vi "Autonomous Independent.vi"   [LabVIEW 2023]
doc: "This VI is called when autonomous begins, and will automatically be terminated when autonomous ends. You can carry out timed or sensor driven robot movement independently without needing to return to the caller."
uses:
  Auto states.ctl
  <vilib>/Rock Robotics/WPI/ThirdParty/REV Robotics/REVLib/Typedef/Spark MAX Idle Mode.ctl
  <vilib>/Rock Robotics/WPI/Utilities/WPI_GetSetVariantRefNum.vi
  <vilib>/Rock Robotics/Network Tables/NT Read String.vi
  <vilib>/Rock Robotics/Network Tables/NT Write Numeric Array.vi
  <vilib>/Rock Robotics/WPI/RobotDrive/WPI_RobotDriveArcadeDrive_Standard(NoSaturation).vi
panel:
  # "Be sure to right-click and choose Data Operations>>Make Current Value default if you want to save the array values with the VI"
types:
  T1 = typedef "WPI_JoystickDevRef.ctl" = cluster{"Device":T2}
  T2 = typedef "WPI_JoystickDeviceEnum.ctl" = enum16{"USB 0", "USB 1", "USB 2", "USB 3", "USB 4", "USB 5"}
  T3 = typedef "Auto states.ctl" = enum16{"Aim", "Fire", "Cross Line", "Pickup", "Reverse Intake", "Return", "Aim 2", "Fire 2", "End"}
  T4 = typedef "Spark MAX Idle Mode.ctl" = enum16{"Coast", "Brake"}
  T5 = typedef "WPI_MotorControlDeviceRef.ctl" = cluster{"DeviceStatus":errorcluster, "Type":T6, "PWM":cluster{"PWM Channel":T7, "DeadBand":T8}, "CAN":cluster{"Device Number":u8, "SetOutput VI Ref":variant, "GetOutput VI Ref":variant, "Enable VI Ref":variant, "Disable VI Ref":variant, "Data":variant}, "Invert":bool, "DIO PWM":cluster{"PWM \"Enable\" Channel":T7, "DIOChannel":T9, "PWM Rate":dbl}}
  T6 = typedef "WPI_MotorControlType.ctl" = enum16{"PWM", "CAN", "DIO PWM"}
  T7 = typedef "FPGA_DIOPWMChannel.ctl" = enum8{"PWM 0", "PWM 1", "PWM 2", "PWM 3", "PWM 4", "PWM 5", "PWM 6", "PWM 7", "PWM 8", "PWM 9", "PWM MXP 0", "PWM MXP 1", "PWM MXP 2", "PWM MXP 3", "PWM MXP 4", "PWM MXP 5", "PWM MXP 6", "PWM MXP 7", "PWM MXP 8", "PWM MXP 9", "Invalid"}
  T8 = typedef "WPI_PWMDeadband.ctl" = cluster{"Name":string, "maxPositivePwm":i32, "minPositivePwm":i32, "centerPwm":i32, "maxNegativePwm":i32, "minNegativePwm":i32, "angularRange":u16}
  T9 = typedef "FPGA_DIOChannel.ctl" = enum8{"DIO 0", "DIO 1", "DIO 2", "DIO 3", "DIO 4", "DIO 5", "DIO 6", "DIO 7", "DIO 8", "DIO 9", "DIO MXP 0", "DIO MXP 1", "DIO MXP 2", "DIO MXP 3", "DIO MXP 4", "DIO MXP 5", "DIO MXP 6", "DIO MXP 7", "DIO MXP 8", "DIO MXP 9", "DIO MXP 10", "DIO MXP 11", "DIO MXP 12", "DIO MXP 13", "DIO MXP 14", "DIO MXP 15", "SPI Port CS1", "SPI Port CS2", "SPI Port CS3", "SPI Port MISO", "SPI Port MOSI", "Invalid"}
  T10 = typedef "WPI_RobotDriveDevRef.ctl" = cluster{"DevStatus":errorcluster, "Motors[]":T5[], "Square Inputs":bool, "Max Output":dbl}
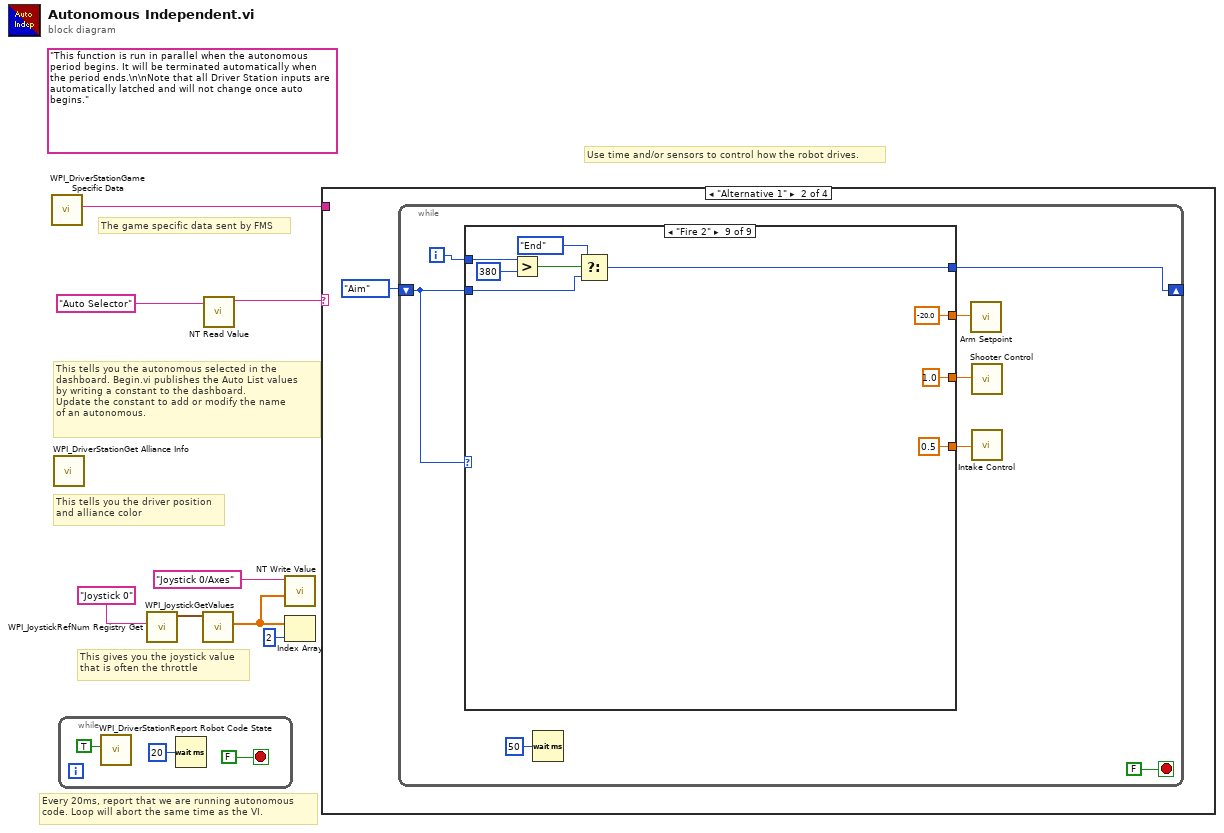
[diagram p0: block diagram]
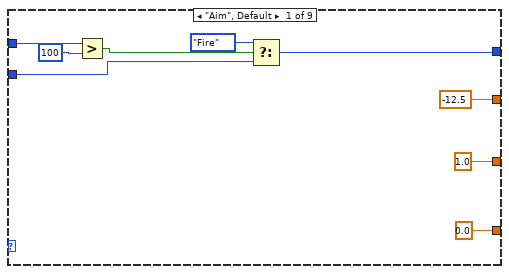
[diagram p3: hidden frame]
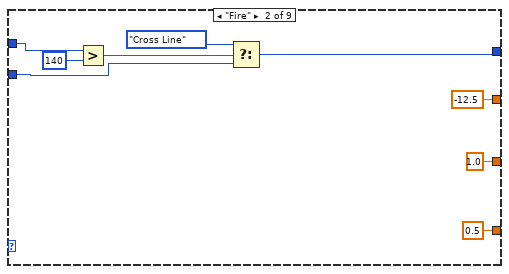
[diagram p4: hidden frame]
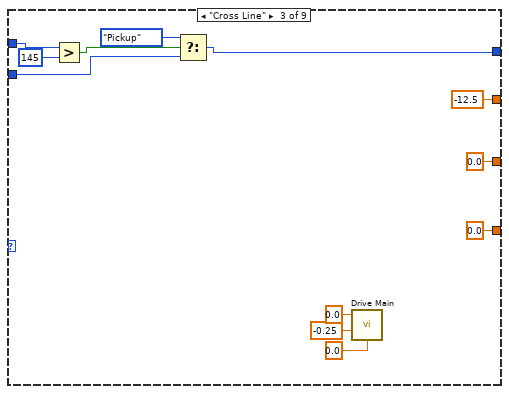
[diagram p5: hidden frame]
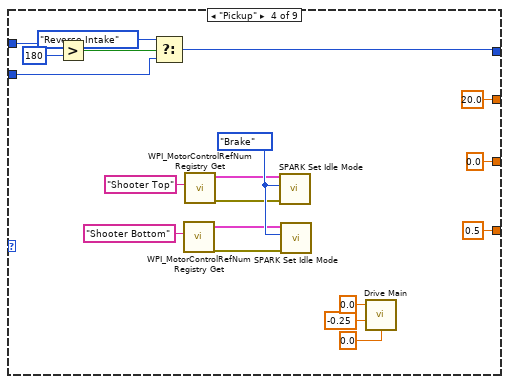
[diagram p6: hidden frame]
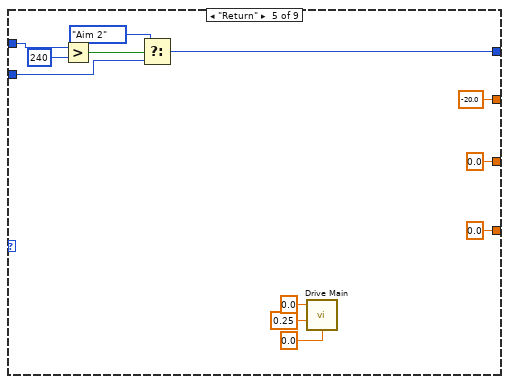
[diagram p7: hidden frame]
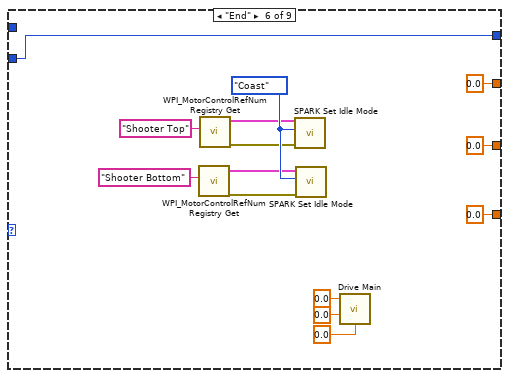
[diagram p8: hidden frame]
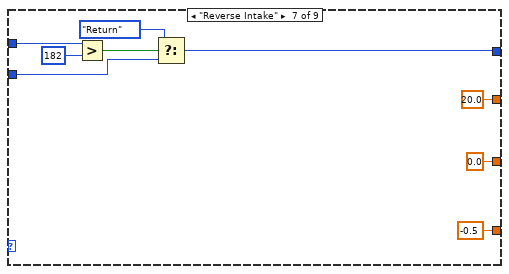
[diagram p9: hidden frame]
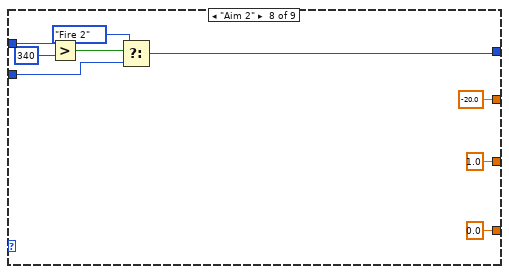
[diagram p10: hidden frame]
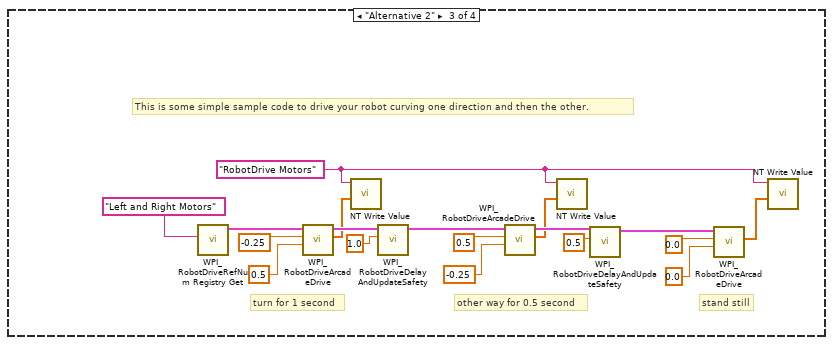
[diagram p11: hidden frame]
diagram:
  (unwired) "This function is run in parallel when the autonomous period begins. It will be terminated automatically when the period ends.\n\nNote that all Driver Station inputs are automatically latched and will not change once auto begins."
  # "The game specific data sent by FMS"
  # "This tells you the autonomous selected in the \ndashboard. Begin.vi publishes the Auto List values\nby writing a constant to the dashboard.\nUpdate the constant to add or modify the name\nof an autonomous."
  # "Every 20ms, report that we are running autonomous\ncode. Loop will abort the same time as the VI."
  # "This gives you the joystick value\nthat is often the throttle"
  # "Use time and/or sensors to control how the robot drives."
  # "This tells you the driver position\nand alliance color"
  n1 = call <vilib>:"WPI_DriverStationGame Specific Data.vi"() -> ("Game Specific Data"=w1:string)  [unwired: 11 in]
  n2 = call <vilib>:"WPI_DriverStationGet Alliance Info.vi"() -> ()  [unwired: 12 out]
  n3 = while {
    stop <- FALSE stop-if-true
    n4 = call <vilib>:"WPI_DriverStationReport Robot Code State.vi"("Autonomous"=TRUE) -> ()  [unwired: 10 in, 1 out]
    n5 = Wait (ms)(milliseconds to wait=u32 20) -> ()  [unwired: 1 out]
  }
  n6 = call <vilib>:"WPI_JoystickRefNum Registry Get.vi"("refnum name"="Joystick 0") -> ("JoystickDevRef"=w7:T1)  [unwired: 1 in, 9 out]
  n7 = call <vilib>:"WPI_JoystickGetValues.vi"("JoystickDevRef"=w7) -> ("Axes"=w3:dbl[])  [unwired: 6 in, 4 out]
  n8 = call-poly <vilib>:"NT Read Value.vi"("name"="Auto Selector" ("Name")) -> ("value"=w4:string)  [unwired: 8 in, 2 out]
  n9 = call-poly <vilib>:"NT Write Value.vi"("value"=w3, "name"="Joystick 0/Axes" ("Name")) -> ()  [unwired: 9 in, 1 out]
  n10 = Index Array(array=w3, index=2) -> ()  [unwired: 1 out]
  n11 = case shown="\"Alternative 1\"" w4 {
    tunnel: w1 -> [_ _ _ _]
    frame Default {
      # "You can put your main auto here, or you can right-click on the case and make any\nother frame be the default case."
      # "This is the frame that will execute if no selection is made, or if it is not recognized"
    }
    frame "Alternative 1" {
      n12 = while {
        shift-right: [w13] -> _
        shift-left: Auto_states."Aim" -> [w14]
        i -> [w15]
        stop <- FALSE stop-if-true
        n13 = case shown="\"Fire 2\"" w14 {
          tunnel: [-12.5 ("Setpoint Angle") -12.5 ("Setpoint Angle") -12.5 ("Setpoint Angle") 20.0 ("Setpoint Angle") -20.0 ("Setpoint Angle") 0.0 ("Setpoint Angle") 20.0 ("Setpoint Angle") -20.0 ("Setpoint Angle") -20.0 ("Setpoint Angle")] -> w18
          tunnel: [1.0 ("Setpoint") 1.0 ("Setpoint") 0.0 ("Setpoint") 0.0 ("Setpoint") 0.0 ("Setpoint") 0.0 ("Setpoint") 0.0 ("Setpoint") 1.0 ("Setpoint") 1.0 ("Setpoint")] -> w17
          tunnel: [0.0 ("Intake Setpoint") 0.5 ("Intake Setpoint") 0.0 ("Intake Setpoint") 0.5 ("Intake Setpoint") 0.0 ("Intake Setpoint") 0.0 ("Intake Setpoint") -0.5 ("Intake Setpoint") 0.0 ("Intake Setpoint") 0.5 ("Intake Setpoint")] -> w16
          tunnel: w15 -> [w26 w35 w47 w66 w78 _ w104 w113 w122]
          tunnel: w14 -> [w23 w32 w44 w63 w75 w95 w101 w110 w119]
          tunnel: [w21 w30 w42 w61 w73 w95 w99 w108 w117] -> w13
          frame "Aim", Default {
            n14 = Greater?(x=w26, y=100) -> (0:w24:bool)
            n15 = Select(t=Auto_states."Fire", s=w24, f=w23) -> (s? t:f=w21:T3)
          }
          frame "Fire" {
            n16 = Greater?(x=w35, y=140) -> (0:w33:bool)
            n17 = Select(t=Auto_states."Cross Line", s=w33, f=w32) -> (s? t:f=w30:T3)
          }
          frame "Cross Line" {
            n18 = Greater?(x=w47, y=145) -> (0:w45:bool)
            n19 = Select(t=Auto_states."Pickup", s=w45, f=w44) -> (s? t:f=w42:T3)
            n20 = call "Drive Main.vi"("spin"=0.0, "In x"=-0.25, "In y"=0.0) -> ()
          }
          frame "Pickup" {
            w55 = Spark_MAX_Idle_Mode."Brake" ("Idle Mode")
            n21 = Greater?(x=w66, y=180) -> (0:w64:bool)
            n22 = Select(t=Auto_states."Reverse Intake", s=w64, f=w63) -> (s? t:f=w61:T3)
            n23 = call <vilib>:"WPI_MotorControlRefNum Registry Get.vi"("refnum name"="Shooter Bottom") -> ("error out"=w51:errorcluster, "MotorControlDevRef"=w54:T5)  [unwired: 9 in]
            n24 = call <vilib>:"WPI_MotorControlRefNum Registry Get.vi"("refnum name"="Shooter Top") -> ("error out"=w52:errorcluster, "MotorControlDevRef"=w53:T5)  [unwired: 9 in]
            n25 = call <vilib>:"SPARK Set Idle Mode.vi"("error in (no error)"=w52, "Idle Mode"=w55, "MotorControlDeviceRef in"=w53) -> ()  [unwired: 7 in, 2 out]
            n26 = call <vilib>:"SPARK Set Idle Mode.vi"("error in (no error)"=w51, "Idle Mode"=w55, "MotorControlDeviceRef in"=w54) -> ()  [unwired: 7 in, 2 out]
            n27 = call "Drive Main.vi"("spin"=0.0, "In x"=-0.25, "In y"=0.0) -> ()
          }
          frame "Return" {
            n28 = Greater?(x=w78, y=240) -> (0:w76:bool)
            n29 = Select(t=Auto_states."Aim 2", s=w76, f=w75) -> (s? t:f=w73:T3)
            n30 = call "Drive Main.vi"("spin"=0.0, "In x"=0.25, "In y"=0.0) -> ()
          }
          frame "End" {
            w86 = Spark_MAX_Idle_Mode."Coast" ("Idle Mode")
            n31 = call <vilib>:"WPI_MotorControlRefNum Registry Get.vi"("refnum name"="Shooter Bottom") -> ("error out"=w82:errorcluster, "MotorControlDevRef"=w85:T5)  [unwired: 9 in]
            n32 = call <vilib>:"WPI_MotorControlRefNum Registry Get.vi"("refnum name"="Shooter Top") -> ("error out"=w83:errorcluster, "MotorControlDevRef"=w84:T5)  [unwired: 9 in]
            n33 = call <vilib>:"SPARK Set Idle Mode.vi"("error in (no error)"=w83, "Idle Mode"=w86, "MotorControlDeviceRef in"=w84) -> ()  [unwired: 7 in, 2 out]
            n34 = call <vilib>:"SPARK Set Idle Mode.vi"("error in (no error)"=w82, "Idle Mode"=w86, "MotorControlDeviceRef in"=w85) -> ()  [unwired: 7 in, 2 out]
            n35 = call "Drive Main.vi"("spin"=0.0, "In x"=0.0, "In y"=0.0) -> ()
          }
          frame "Reverse Intake" {
            n36 = Greater?(x=w104, y=182) -> (0:w102:bool)
            n37 = Select(t=Auto_states."Return", s=w102, f=w101) -> (s? t:f=w99:T3)
          }
          frame "Aim 2" {
            n38 = Greater?(x=w113, y=340) -> (0:w111:bool)
            n39 = Select(t=Auto_states."Fire 2", s=w111, f=w110) -> (s? t:f=w108:T3)
          }
          frame "Fire 2" {
            n40 = Greater?(x=w122, y=380) -> (0:w120:bool)
            n41 = Select(t=Auto_states."End", s=w120, f=w119) -> (s? t:f=w117:T3)
          }
        }
        n42 = Wait (ms)(milliseconds to wait=u32 50) -> ()  [unwired: 1 out]
        n43 = call "Arm Setpoint.vi"("Setpoint Angle"=w18) -> ()  [unwired: 1 in]
        n44 = call "Shooter Control.vi"("Setpoint"=w17) -> ()  [unwired: 1 in]
        n45 = call "Intake Control.vi"("Intake Setpoint"=w16) -> ()  [unwired: 1 in]
      }
    }
    frame "Alternative 2" {
      w124 = "RobotDrive Motors" ("Name")
      # "This is some simple sample code to drive your robot curving one direction and then the other."
      # "stand still"
      # "other way for 0.5 second"
      # "turn for 1 second"
      n46 = call <vilib>:"WPI_RobotDriveRefNum Registry Get.vi"("refnum name"="Left and Right Motors") -> ("RobotDriveDevRef"=w140:T10)  [unwired: 1 in, 9 out]
      n47 = call-poly <vilib>:"WPI_RobotDriveArcadeDrive.vi"("Y axis value"=0.5 ("X axis value"), "X axis value"=-0.25, "RobotDriveDevRef"=w140) -> ("Motor Values"=w123:dbl[], "RobotDriveDevRef"=w133:T10)  [unwired: 1 in, 6 out]
      n48 = call-poly <vilib>:"NT Write Value.vi"("value"=w123, "name"=w124) -> ()  [unwired: 9 in, 1 out]
      n49 = call <vilib>:"WPI_RobotDriveDelayAndUpdateSafety.vi"("Delay (s)"=1.0, "RobotDriveDevRef"=w133) -> ("RobotDriveDevRef 2"=w134:T10)  [unwired: 8 in, 1 out]
      n50 = call-poly <vilib>:"WPI_RobotDriveArcadeDrive.vi"("Y axis value"=-0.25 ("X axis value"), "X axis value"=0.5, "RobotDriveDevRef"=w134) -> ("Motor Values"=w125:dbl[], "RobotDriveDevRef"=w135:T10)  [unwired: 1 in, 6 out]
      n51 = call-poly <vilib>:"NT Write Value.vi"("value"=w125, "name"=w124) -> ()  [unwired: 9 in, 1 out]
      n52 = call <vilib>:"WPI_RobotDriveDelayAndUpdateSafety.vi"("Delay (s)"=0.5, "RobotDriveDevRef"=w135) -> ("RobotDriveDevRef 2"=w136:T10)  [unwired: 8 in, 1 out]
      n53 = call-poly <vilib>:"WPI_RobotDriveArcadeDrive.vi"("Y axis value"=0.0 ("X axis value"), "X axis value"=0.0, "RobotDriveDevRef"=w136) -> ("Motor Values"=w126:dbl[])  [unwired: 1 in, 7 out]
      n54 = call-poly <vilib>:"NT Write Value.vi"("value"=w126, "name"=w124) -> ()  [unwired: 9 in, 1 out]
    }
    frame "Your Turn" {
    }
  }
